vi "read offsets.vi"(8 "error in (no error)":errorcluster, 11 "offsets.ini path":path) -> (0 "error out":errorcluster, 2 "offsets":T1)   [LabVIEW 2017, in "DAQ.lvclass"]
doc: "Developed by Kevin Thompson\nkevin@thompsonengineering.net\n\nCopyright 2018-2020\nThompson Engineering, LLC"
uses:
  DAQ.lvclass
  DataTypes/offsets cluster.ctl
  <vilib>/Utility/config.llb/NI_LVConfig.lvlib
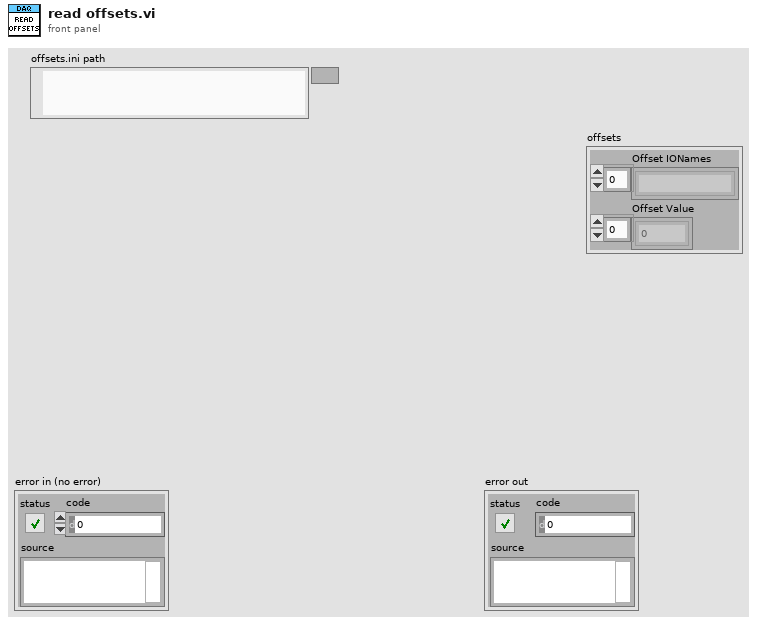
[diagram p1: front panel]
types:
  T1 = typedef "DAQ.lvclass/offsets cluster.ctl" = cluster{"Offset IONames":string[], "Offset Value":dbl[]}
  T2 = typedef "NI_LVConfig.lvlib/Config Data RefNum.ctl" = refnum<k1>
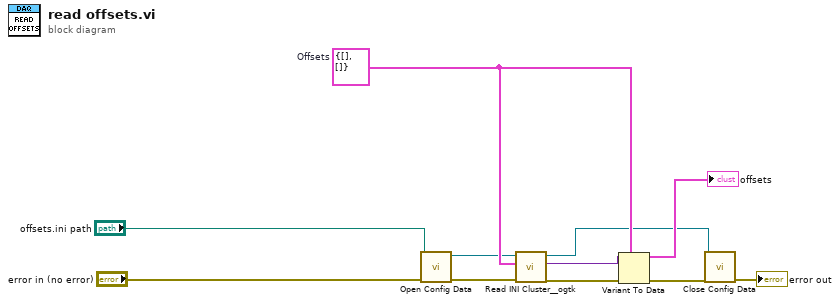
[diagram p0: block diagram]
diagram:
  w8 = T1 {"Offset IONames"=[], "Offset Value"=[]}  # Offsets
  n1 = call <vilib>:"Open Config Data.vi"("error in (no error)"="error in (no error)", "configuration file path"="offsets.ini path") -> ("error out"=w2:errorcluster, "refnum"=w6:T2)  [unwired: 7 in, 1 out]
  n2 = call <userlib>:"Read INI Cluster__ogtk.vi"("error in (no error)"=w2, "INI Fomatted Cluster Type"=w8, "refnum"=w6) -> ("error out"=w3:errorcluster, "INI Fomatted Cluster"=w9:variant, "dup refnum"=w5:T2)  [unwired: 4 in, 2 out]
  n3 = Variant To Data(error in=w3, type=w8, Variant=w9) -> (data=→"offsets":T1, error out=w4:errorcluster)
  n4 = call <vilib>:"Close Config Data.vi"("error in (no error)"=w4, "refnum"=w5) -> ("error out"=→"error out":errorcluster)  [unwired: 8 in, 1 out]
